vi "以众电机控制.vi"() -> ()   [LabVIEW 2018]
uses:
  Device VIs/Verbal.vi
  <vilib>/Instr/_visa.llb/VISA Configure Serial Port (Instr).vi
panel:
  out "当前位置":i32[](array[numeric])
  in  "小平台X限位":dbl=3000.0 caption="小平台X轴限位/um" min=-8388607.0 max=8388607.0
  in  "设置坐标":bool caption="X jog"
  in  "开始连接":bool
  out "状态":string
  out "执行":bool
  out "OK":bool
  in  "电机":T1(ring)
  in  "结束":bool
  in  "制动":bool
  out "位置信息":i32(listbox)
  out "pic3Left":bool caption="0位"
  out "pic3Right":bool caption="限位"
  out "pic2Left":bool caption="0位"
  out "pic2Right":bool caption="限位"
  out "pic1Left":bool caption="0位"
  out "pic1Right":bool caption="限位"
  out "Z Left":bool caption="0位"
  out "Z Right":bool caption="限位"
  out "Y Left":bool caption="0位"
  out "Y Right":bool caption="限位"
  out "X Lift":bool caption="0位"
  out "X Right":bool caption="限位"
  in  "连续反转":bool
  in  "坐标移动":bool caption="X jog"
  out "设定位置":i32
  in  "坐标":enum16{"位置0", "位置1", "位置2", "位置3"}(ring) caption="位置"
  in  "连续正转":bool
  in  "归0":bool
  in  "启动":bool
  in  "Step":dbl caption="步进\n um" min=-8388607.0 max=8388607.0
  # "电机"
  # "大平台X"
  # "大平台Y"
  # "大平台Z"
  # "小平台X"
  # "小平台Y"
  # "小平台Z"
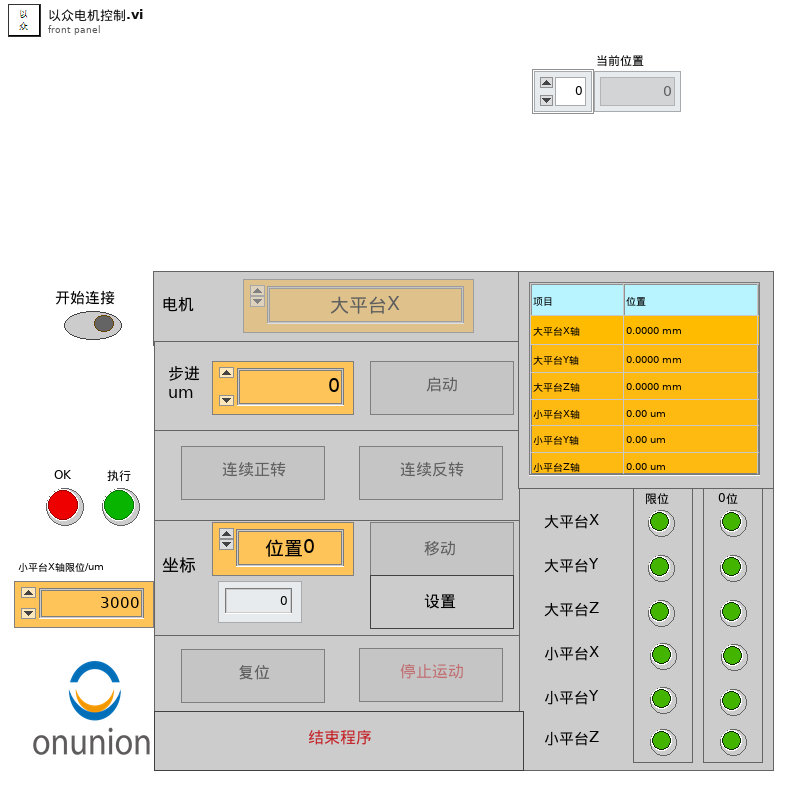
[diagram p1: front panel]
types:
  T1 = enum16{"大平台X", "大平台Y", "大平台Z", "小平台X", "小平台Y", "小平台Z"}
  T2 = enum8{"Enabled", "Disabled", "Disabled and Grayed Out"}
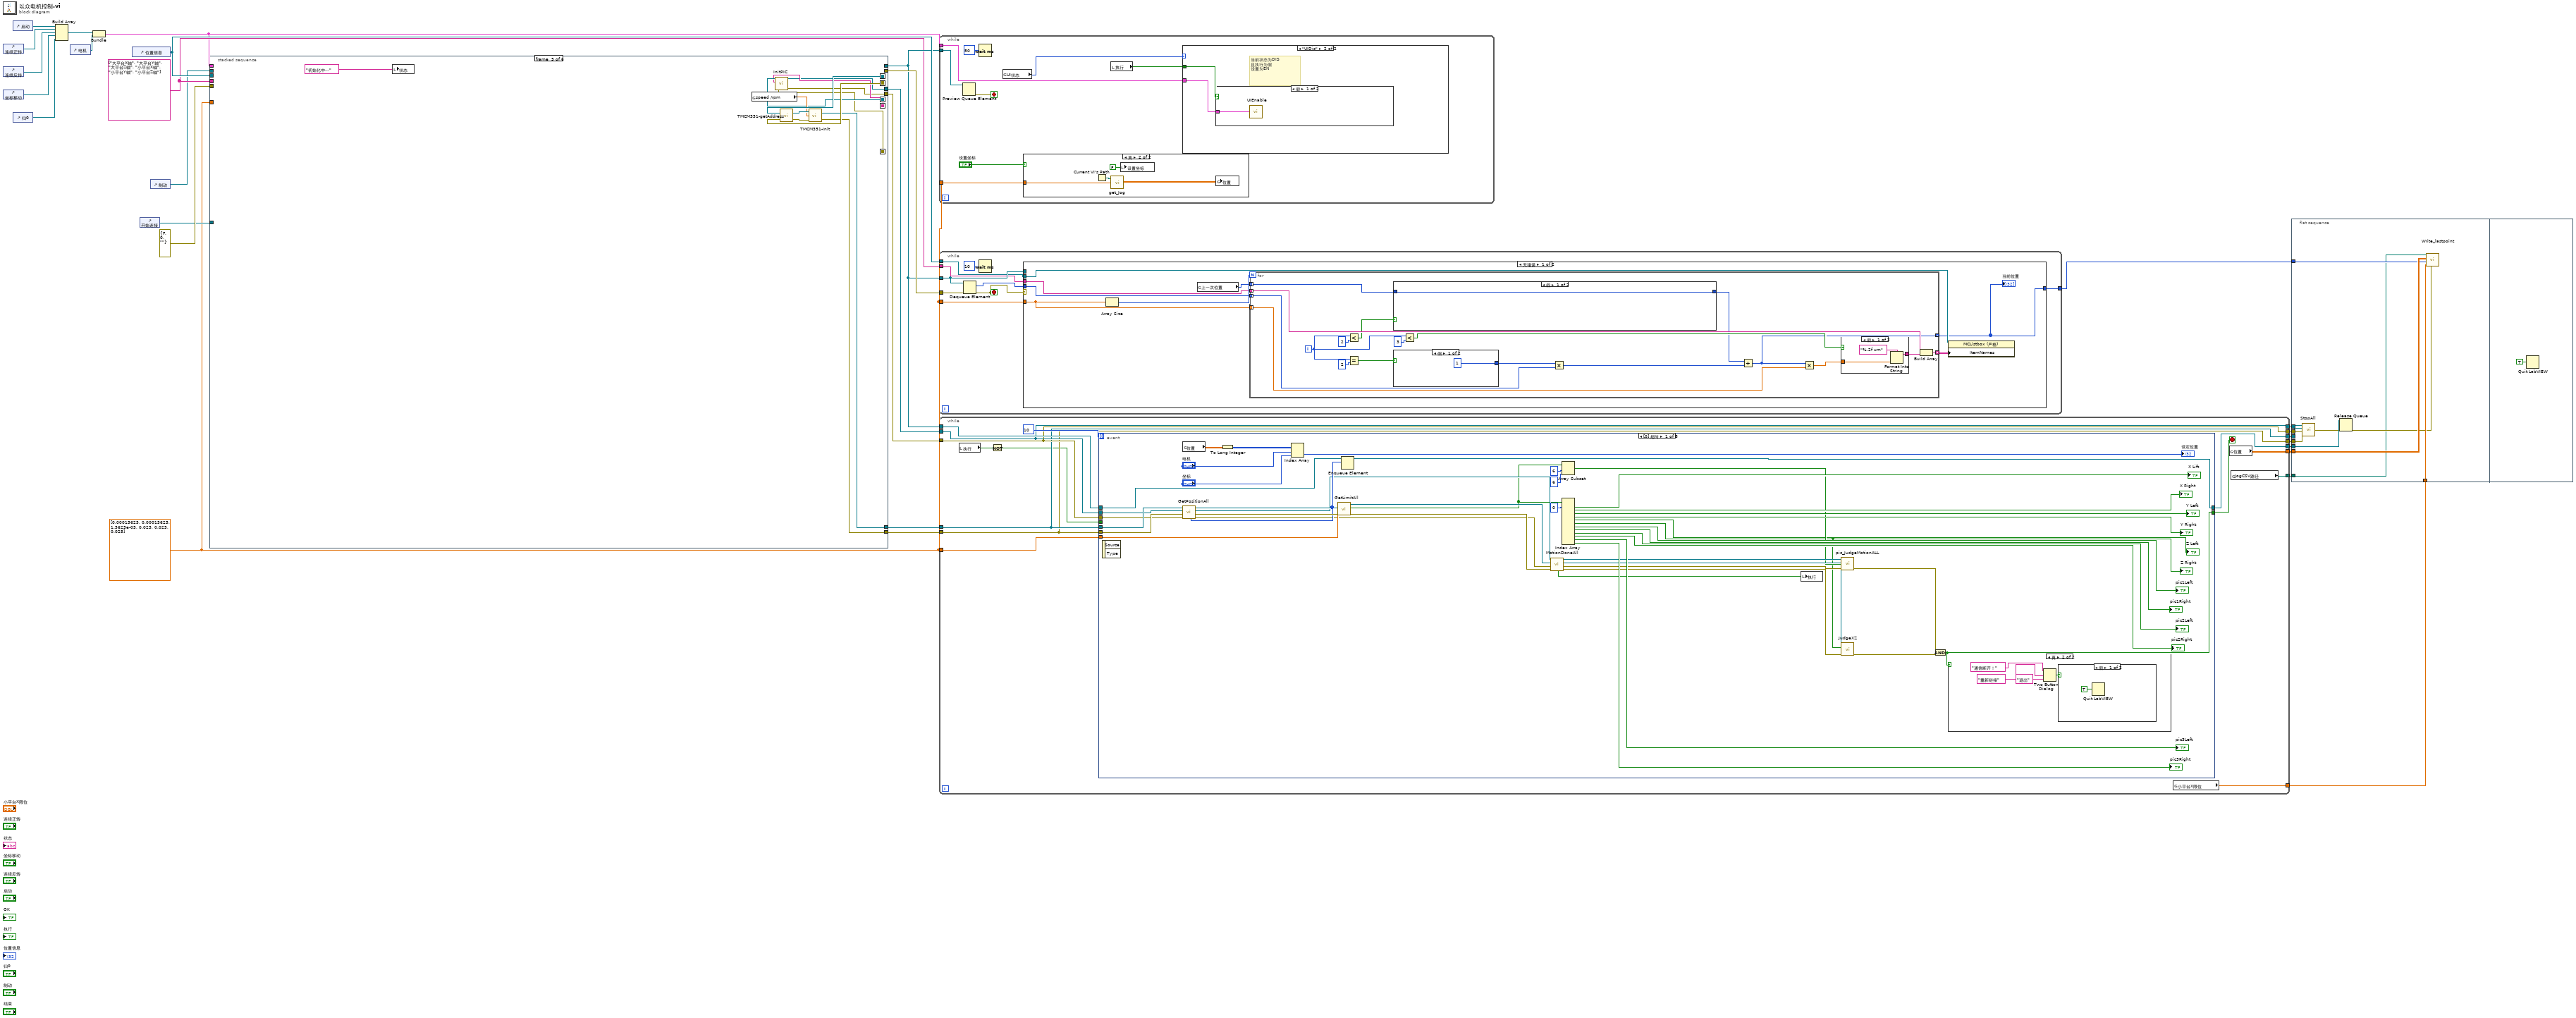
[diagram p0: block diagram]
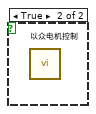
[diagram p3: hidden frame]
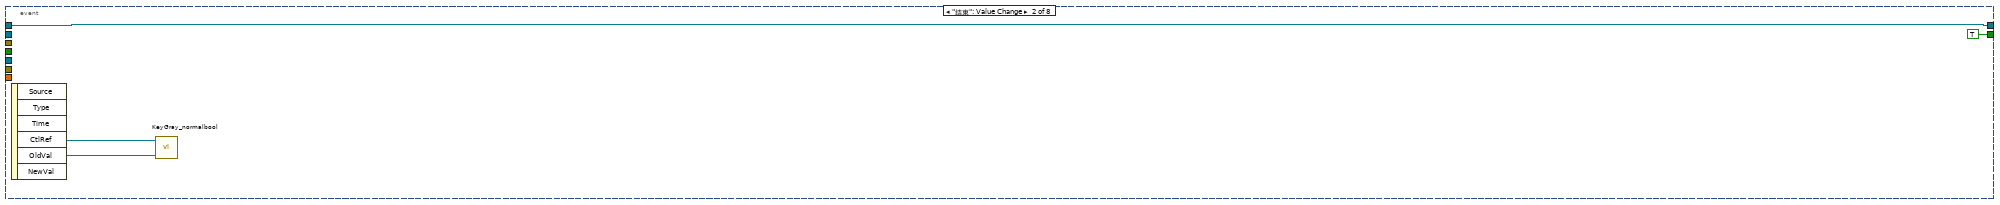
[diagram p4: hidden frame]
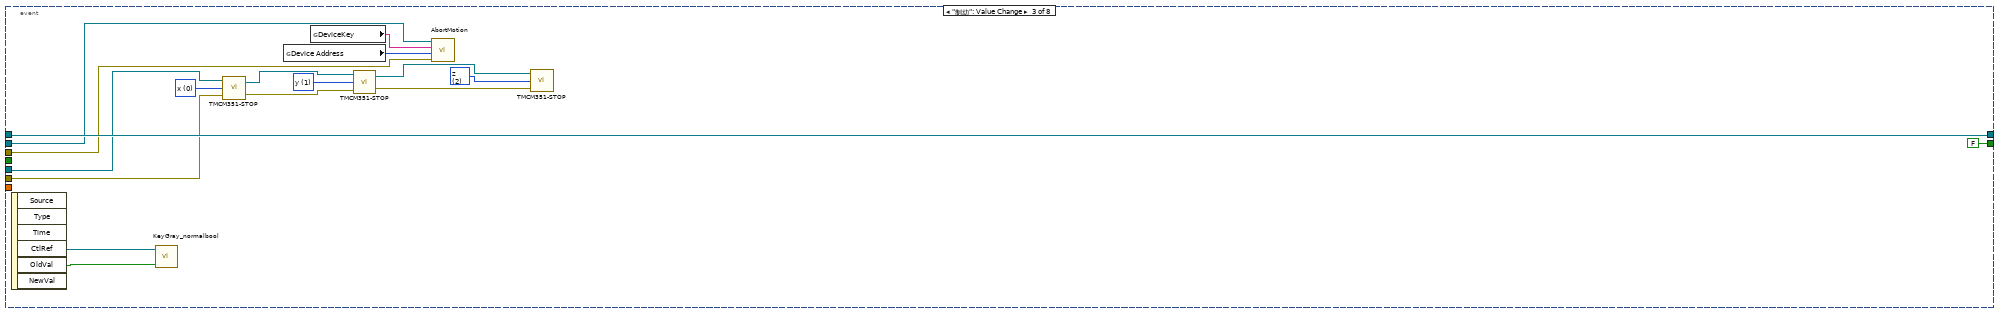
[diagram p5: hidden frame]
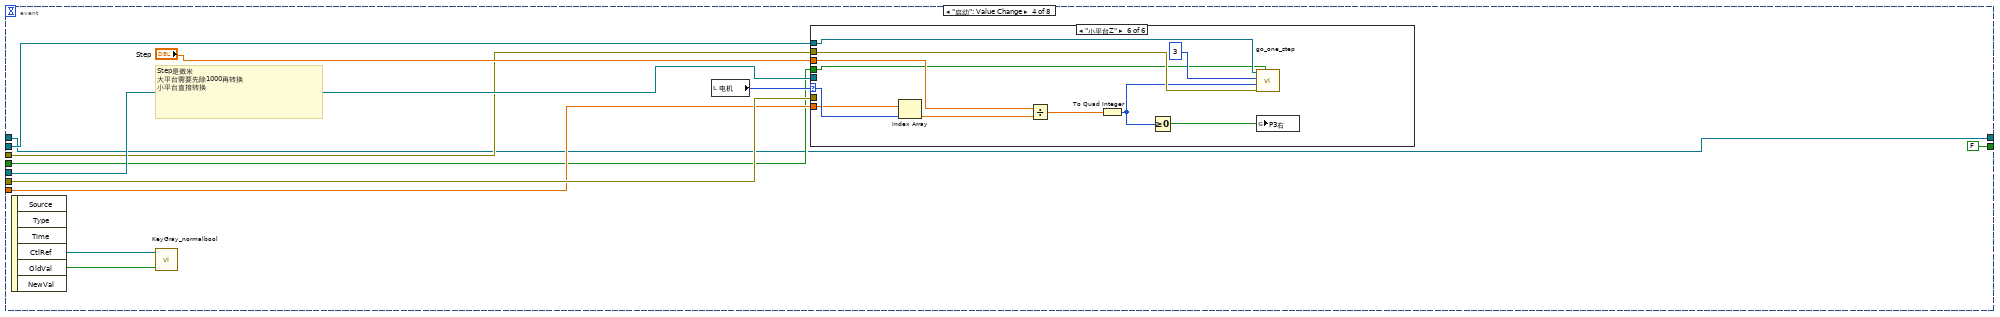
[diagram p6: hidden frame]
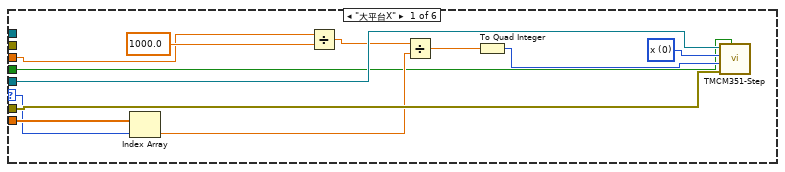
[diagram p7: hidden frame]
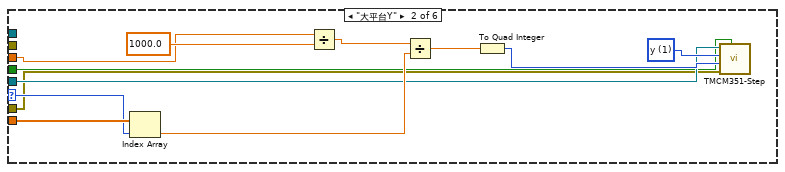
[diagram p8: hidden frame]
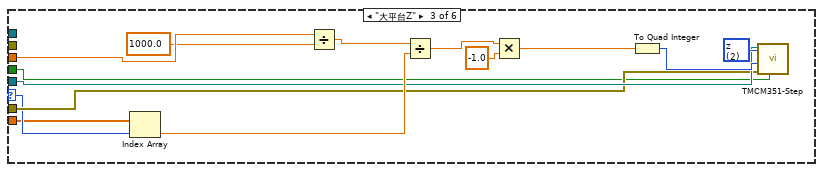
[diagram p9: hidden frame]
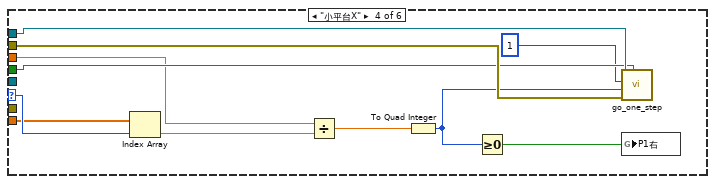
[diagram p10: hidden frame]
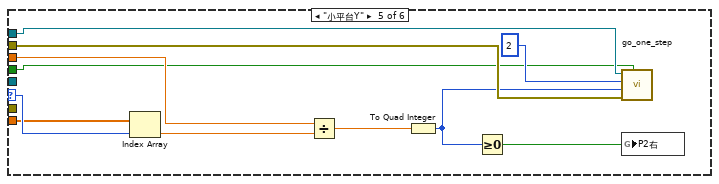
[diagram p11: hidden frame]
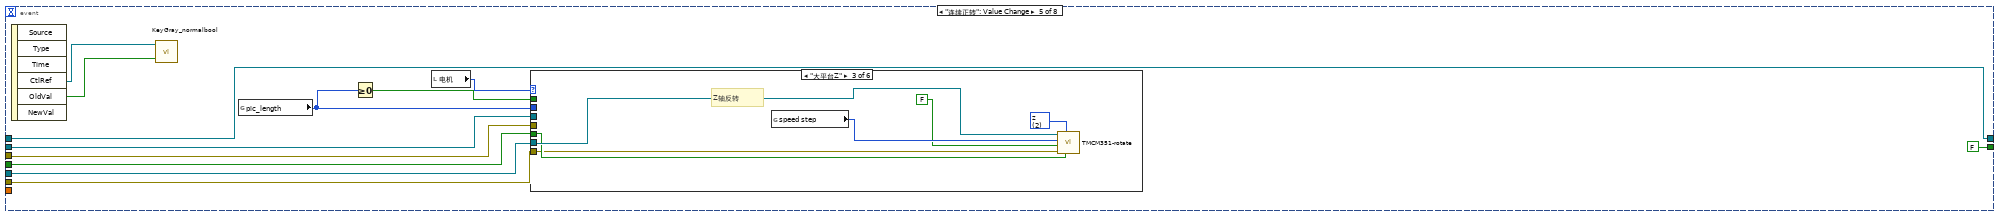
[diagram p12: hidden frame]
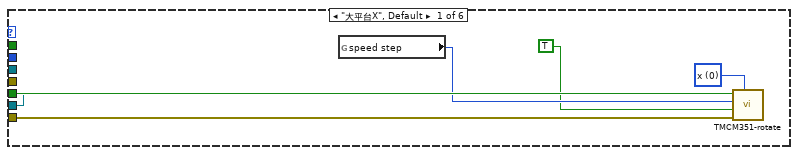
[diagram p13: hidden frame]
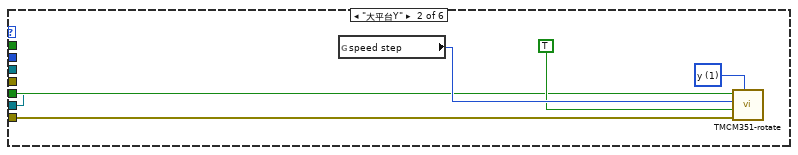
[diagram p14: hidden frame]
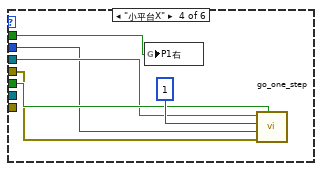
[diagram p15: hidden frame]
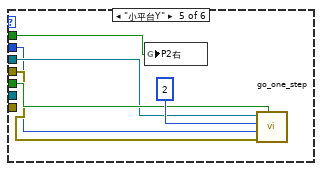
[diagram p16: hidden frame]
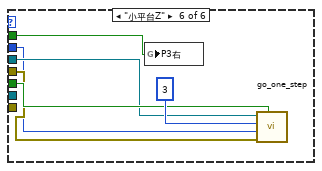
[diagram p17: hidden frame]
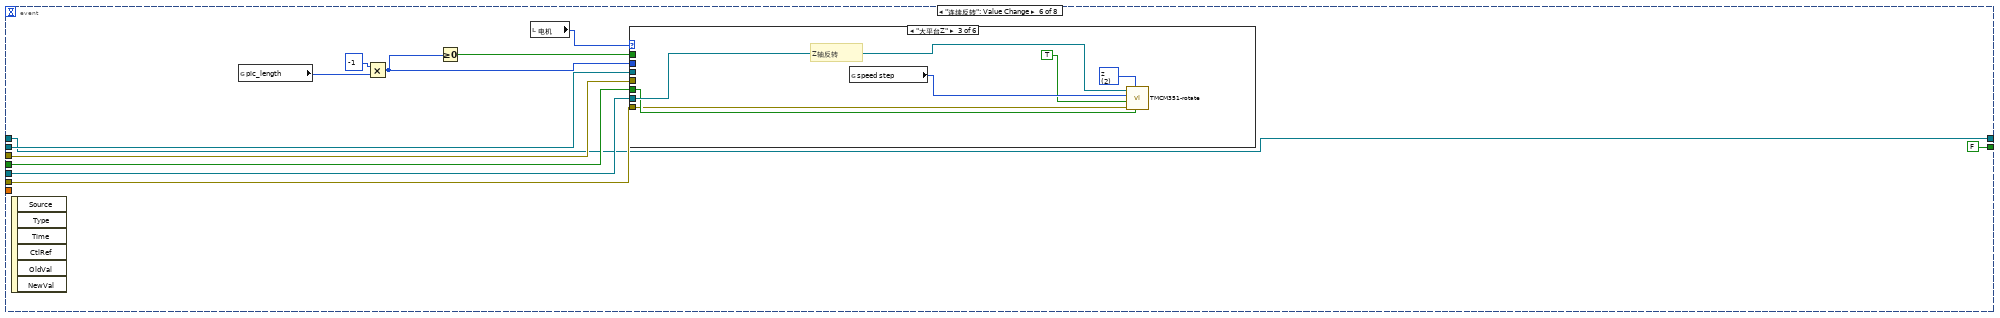
[diagram p18: hidden frame]
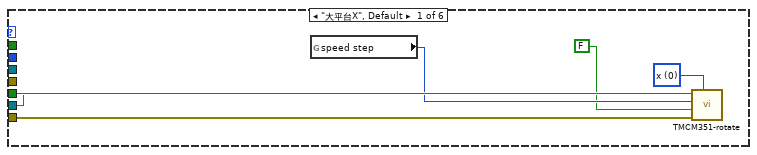
[diagram p19: hidden frame]
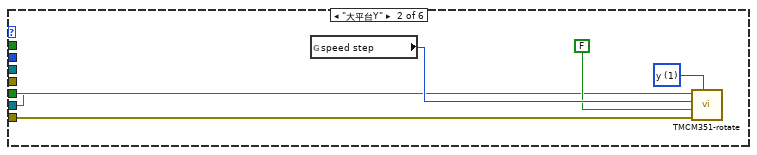
[diagram p20: hidden frame]
diagram:
  w7 = string[] ["大平台X轴", "大平台Y轴", "大平台Z轴", "小平台X轴", "小平台Y轴", "小平台Z轴"]
  w16 = dbl[] [0.00015625, 0.00015625, 1.5625e-05, 0.025, 0.025, 0.025]
  n1 = control-ref of="连续正转"() -> (w27:refnum<vi>)
  n2 = control-ref of="连续反转"() -> (w26:refnum<vi>)
  n3 = control-ref of="坐标移动"() -> (w25:refnum<vi>)
  n4 = control-ref of="启动"() -> (w28:refnum<vi>)
  n5 = control-ref of="归0"() -> (w24:refnum<vi>)
  n6 = Build Array(w28, w27, w26, w25, w24) -> (w4:refnum<vi>[])
  n7 = control-ref of="电机"() -> (w3:refnum<vi>)
  n8 = Bundle(w4, "电机"=w3) -> (w2:cluster{refnum<vi>[], "电机":refnum<vi>})  [unwired: 1 in]
  n9 = control-ref of="位置信息"() -> (w22:refnum<vi>)
  n10 = control-ref of="开始连接"() -> (w23:refnum<vi>)
  n11 = control-ref of="制动"() -> (w6:refnum<vi>)
  n12 = stacked-sequence {
    seq-local: [_ _ _ w75 _ _] -> [_ _ _ _ w107 _]
    seq-local: [_ _ _ w76 _ _] -> [_ _ _ _ w108 _]
    seq-local: [_ _ _ w74 _ _] -> [_ _ _ _ w102 _]
    seq-local: [_ _ _ w73 _ _] -> [_ _ _ _ w101 _]
    seq-local: [_ _ _ w72 _ _] -> [_ _ _ _ w103 _]
    tunnel: w16 -> [_ w46 _ _ _ _]
    tunnel: errorcluster {"status"=FALSE, "code"=0, "source"=""} ("error in (no error)") -> [_ w63 _ w83 _ _]
    tunnel: w22 -> [_ w55 _ _ _ _]
    tunnel: w7 -> [_ w58 _ _ _ _]
    tunnel: w23 -> [w34 _ _ _ _ w121]
    tunnel: [_ _ _ _ w100 _] -> w18
    tunnel: [_ _ _ _ w99 _] -> w17
    tunnel: [_ _ _ _ w98 _] -> w20
    tunnel: [_ _ _ _ w97 _] -> w19
    tunnel: [_ _ _ _ _ w115] -> w8
    tunnel: [_ _ _ _ _ w114] -> w21
    tunnel: w6 -> [w32 _ _ _ _ w112]
    tunnel: w2 -> [w30 _ _ _ _ w110]
    frame #0 {
      n13 = call "UIDisable.vi"("引用簇"=w30) -> ()  [unwired: 1 in]
      n14 = property class="Bool (严格)"(reference=w34, "DisabledEnum"=T2."Enabled" ("禁用")) -> ()  [unwired: 1 in, 2 out]
      n15 = property class="Bool (严格)"(reference=w32, "DisabledEnum"=T2."Disabled and Grayed Out" ("禁用")) -> ()  [unwired: 1 in, 2 out]
    }
    frame #1 {
      w37 = FALSE
      w36 = FALSE
      w38 = FALSE
      w40 = FALSE
      n16 = Current VI's Path() -> (path=w64:path)
      n17 = Array Size(array=w58) -> (size(s)=w57:i32)
      n18 = Index Array(array=w46, index=3 ("索引")) -> (element=w44:dbl)
      n19 = call "get_Jog.vi"("error in (no error)"=w63, "坐标转换"=w46, "路径"=w64) -> ("上次限位"=w35:dbl, "当前位置"=w59:string[], "坐标位置"=w48:dbl[][], "上一次位置"=w47:i32[], "File Out"=w39:path)  [unwired: 1 out]
      n20 = local write "执行"(FALSE ("执行")) -> ()
      n21 = local write "OK"(FALSE ("OK")) -> ()
      n22 = global write "Verbal.vi" "speed /rpm"(10 ("speed step")) -> ()
      n23 = global write "Verbal.vi" "acc pic"(10000 ("acc pic")) -> ()
      n24 = global write "Verbal.vi" "px0?"(w40) -> ()
      n25 = global write "Verbal.vi" "py0?"(w40) -> ()
      n26 = global write "Verbal.vi" "pz0?"(w40) -> ()
      n27 = global write "Verbal.vi" "xz0?"(w40) -> ()
      n28 = local write "Z Left"(w37) -> ()
      n29 = local write "pic1Left"(w37) -> ()
      n30 = local write "pic2Left"(w37) -> ()
      n31 = local write "pic3Left"(w37) -> ()
      n32 = local write "pic2Right"(w36) -> ()
      n33 = local write "pic3Right"(w36) -> ()
      n34 = local write "X Lift"(w36) -> ()
      n35 = local write "Y Left"(w36) -> ()
      n36 = local write "开始连接"(w36) -> ()
      n37 = local write "设置坐标"(w36) -> ()
      n38 = local write "X Right"(w38) -> ()
      n39 = local write "Y Right"(w38) -> ()
      n40 = local write "Z Right"(w38) -> ()
      n41 = local write "pic1Right"(w38) -> ()
      n42 = global write "Verbal.vi" "speed pic"(1000 ("speed pic")) -> ()
      n43 = Build Array("项目", "位置") -> (w62:string[])
      n44 = property on="属性节点" class="MCListbox (严格)"(reference=w55, "ColHdrString"=w62) -> ()  [unwired: 1 in, 2 out]
      n45 = global write "Verbal.vi" "位置"(w48) -> ()
      n46 = global write "Verbal.vi" "上一次位置"(w47) -> ()
      n47 = global write "Verbal.vi" "JogCSV路径"(w39) -> ()
      n48 = global write "Verbal.vi" "小平台X限位"(w35) -> ()
      n49 = local write "小平台X限位"(w35) -> ()
      n50 = for {
        N: w57 -> [_]
        tunnel: w59 -> [w65] mode=indexing
        tunnel: w58 -> [w66] mode=indexing
        tunnel: [w67] -> w56 mode=indexing
        n51 = Build Array(w66, w65) -> (w67:string[])
      }
      n52 = Divide(x=15000.0, y=w44) -> (x/y=w42:dbl)
      n53 = local write "状态"("请点击开始连接" ("状态")) -> ()
      n54 = To Long Integer(number=w42) -> (32bit integer=w41:i32)
      n55 = global write "Verbal.vi" "pic_length"(w41) -> ()
      n56 = property on="属性节点" class="MCListbox (严格)"(reference=w55, "ItemNames"=w56) -> ()  [unwired: 1 in, 2 out]
    }
    frame #2 {
      n57 = flat-sequence {
        frame #0 {
          n58 = while {
            stop <- "开始连接" stop-if-true
            n59 = local read "结束"() -> (w68:bool)
            n60 = Wait (ms)(milliseconds to wait=u32 20 ("等待时间（毫秒）")) -> ()  [unwired: 1 out]
            n61 = Quit LabVIEW(quit? (T)=w68) -> ()
          }
        }
        frame #1 {
          n62 = local write "状态"("查找设备中...." ("状态")) -> ()
        }
      }
    }
    frame #3 {
      n63 = call "InitSingleDevice.vi"("error in (no error)"=w83, "msecDelayForDiscovery"=1000) -> ("error out"=w73:errorcluster, "DeviceKey Out"=w74:string, "CmdLib Out"=w72:refnum<k24>)  [unwired: 3 in]
      n64 = call "findCOM.vi"("error in (no error)"=w83) -> ("错误输出"=w85:errorcluster, "VISA resource out"=w86:refnum<visa-resource-name>)  [unwired: 1 in]
      n65 = String Length(string=w74) -> (length=w82:i32)
      n66 = call-poly "VISA Configure Serial Port"("VISA resource name"=w86, "Enable Termination\nChar (T)"=FALSE ("Enable Termination\nChar (T)"), "baud rate (9600)"=u32 115200, "error in (no error)"=w85) -> ("VISA resource name out"=w79:refnum<visa-resource-name>, "error out"=w78:errorcluster)  [unwired: 10 in]
      n67 = property class="Instr"(reference=w79, error in=w78) -> (reference out=w75:refnum<visa-resource-name>, error out=w76:errorcluster, "Intf Num"=w77:u16)
      n68 = Equal To 0?(x=w82) -> (x = 0?=w81:bool)
      n69 = And(x=w76, y=w81) -> (x .and. y?=w80:bool)
      n70 = case shown="真" w80 {
        tunnel: w74 -> [_ w94]
        tunnel: w77 -> [_ w93]
        frame False {
        }
        frame True {
          n71 = Format Into String(format string="请检查通信和电源\\nCOM:%d;PIC:%s" ("格式字符串"), w93, w94) -> (resulting string=w92:string)  [unwired: 2 in, 1 out]
          n72 = Two Button Dialog(message=w92, 1:"退出" ("F按钮名称（“取消”）"), 2:"重新链接" ("T按钮名称（“确定”）")) -> (T button?=w89:bool)
          n73 = case shown="假" w89 {
            frame False {
              n74 = Quit LabVIEW(quit? (T)=TRUE ("停止？(T)")) -> ()
            }
            frame True {
              n75 = call "以众电机控制.vi"() -> ()  [unwired: 12 in]
            }
          }
        }
      }
    }
    frame #4 {
      n76 = local write "状态"("初始化中..." ("状态")) -> ()
      n77 = global read "Verbal.vi" "speed /rpm"() -> (w104:dbl)
      n78 = call "InitPIC.vi"("error in (no error)"=w101, "DeviceKey In"=w102, "CmdLib In"=w103) -> ("error out"=w99:errorcluster, "CmdLib Out"=w100:refnum<k24>)  [unwired: 1 in, 2 out]
      n79 = call "TMCM351-getAddress.vi"("错误输入"=w108, "com in"=w107) -> ("错误输出"=w105:errorcluster, "com out"=w106:refnum<visa-resource-name>)
      n80 = call "TMCM351-Init.vi"("错误输入"=w105, "Speed /rpm"=w104, "com in"=w106) -> ("错误输出"=w97:errorcluster, "com out"=w98:refnum<visa-resource-name>)
    }
    frame #5 {
      n81 = call "UIEnable.vi"("引用簇"=w110) -> ()  [unwired: 1 in]
      n82 = local write "OK"(TRUE ("OK")) -> ()
      n83 = local write "执行"(FALSE ("执行")) -> ()
      n84 = local write "状态"("欢迎使用" ("状态")) -> ()
      n85 = property class="Bool (严格)"(reference=w112, "DisabledEnum"=T2."Enabled" ("禁用")) -> ()  [unwired: 1 in, 2 out]
      n86 = property class="Bool (严格)"(reference=w121, "DisabledEnum"=T2."Disabled and Grayed Out" ("禁用")) -> ()  [unwired: 1 in, 2 out]
      n87 = Obtain Queue(name (unnamed)="位置消息" ("名称（未命名）"), element data type=i32[] []) -> (queue out=w115:refnum<queue>, error out=w114:errorcluster)  [unwired: 3 in, 1 out]
    }
  }
  n88 = while {
    tunnel: w16 -> [w127]
    tunnel: w2 -> [w124]
    tunnel: w8 -> [w123]
    stop <- w122 stop-if-true
    n89 = Preview Queue Element(queue=w123) -> (error out=w122:errorcluster)  [unwired: 2 in, 3 out]
    n90 = Wait (ms)(milliseconds to wait=u32 50 ("等待时间（毫秒）")) -> ()  [unwired: 1 out]
    n91 = global read "Verbal.vi" "UI状态"() -> (w126:enum16{"UIEn", "UIDis"})
    n92 = case shown="真" "设置坐标" {
      tunnel: w127 -> [_ w137]
      frame False {
      }
      frame True {
        n93 = Current VI's Path() -> (path=w138:path)
        n94 = call "get_Jog.vi"("坐标转换"=w137, "路径"=w138) -> ("坐标位置"=w136:dbl[][])  [unwired: 1 in, 5 out]
        n95 = local write "设置坐标"(FALSE ("设置坐标")) -> ()
        n96 = global write "Verbal.vi" "位置"(w136) -> ()
      }
    }
    n97 = local read "执行"() -> (w125:bool)
    n98 = case shown="\"UIDis\"" w126 {
      tunnel: w124 -> [w131 w134]
      tunnel: w125 -> [w130 w133]
      frame "UIEn", Default {
        # "当前状态为EN\n且执行为真\n设置为Dis"
        n99 = case shown="真" w130 {
          tunnel: w131 -> [_ w132]
          frame False {
          }
          frame True {
            n100 = call "UIDisable.vi"("引用簇"=w132) -> ()  [unwired: 1 in]
          }
        }
      }
      frame "UIDis" {
        # "当前状态为DIS\n且执行为假\n设置为EN"
        n101 = case shown="假" w133 {
          tunnel: w134 -> [w135 _]
          frame False {
            n102 = call "UIEnable.vi"("引用簇"=w135) -> ()  [unwired: 1 in]
          }
          frame True {
          }
        }
      }
    }
  }
  n103 = while {
    tunnel: w8 -> [w148]
    tunnel: w21 -> [w141]
    tunnel: w16 -> [w147]
    tunnel: w7 -> [w146]
    tunnel: w22 -> [w145]
    tunnel: [w144] -> w5
    stop <- w140 stop-if-true
    n104 = Dequeue Element(queue=w148, error in (no error)=w141) -> (element=w142:i32[], error out=w140:errorcluster)  [unwired: 1 in, 2 out]
    n105 = Wait (ms)(milliseconds to wait=u32 10 ("等待时间（毫秒）")) -> ()  [unwired: 1 out]
    n106 = case shown="无错误" w140 {
      tunnel: w148 -> [_ _]
      tunnel: w147 -> [w156 _]
      tunnel: w146 -> [w154 _]
      tunnel: w145 -> [w152 _]
      tunnel: [w149 w185] -> w144
      tunnel: w142 -> [w150 _]
      frame No Error {
        n107 = Array Size(array=w156) -> (size(s)=w155:i32)
        n108 = global read "Verbal.vi" "上一次位置"() -> (w151:i32[])
        n109 = for {
          N: w155 -> [_]
          tunnel: w156 -> [w174] mode=indexing
          tunnel: w154 -> [w171] mode=indexing
          tunnel: [w169] -> w153 mode=indexing
          tunnel: w151 -> [w166] mode=indexing
          tunnel: [w165] -> w149 mode=indexing
          tunnel: w150 -> [w159] mode=indexing
          i -> [w164]
          n110 = Less?(x=w164, y=2) -> (x < y?=w167:bool)
          n111 = Equal?(x=w164, y=2) -> (x = y?=w161:bool)
          n112 = case shown="假" w167 {
            tunnel: [w177 0] -> w157
            tunnel: w166 -> [w177 _]
            frame False {
            }
            frame True {
              # "小于2是大平台XY\n已经写入了不用修正"
            }
          }
          n113 = case shown="假" w161 {
            tunnel: [1 -1] -> w162
            frame False {
            }
            frame True {
            }
          }
          n114 = Less?(x=w164, y=3) -> (x < y?=w172:bool)
          n115 = Multiply(x=w162, y=w159) -> (x*y=w158:i32)
          n116 = Add(x=w157, y=w158) -> (x+y=w165:i32)
          n117 = Multiply(x=w165, y=w174) -> (x*y=w160:dbl)
          n118 = case shown="假" w172 {
            tunnel: w160 -> [w179 w182]
            tunnel: [w180 w183] -> w170
            frame False {
              n119 = Format Into String(format string="%.2f um" ("格式字符串"), w179) -> (resulting string=w180:string)  [unwired: 2 in, 1 out]
            }
            frame True {
              n120 = Format Into String(format string="%.4f mm" ("格式字符串"), w182) -> (resulting string=w183:string)  [unwired: 2 in, 1 out]
            }
          }
          n121 = Build Array(w171, w170) -> (w169:string[])
        }
        "当前位置" <- w149
        n122 = property on="属性节点" class="MCListbox (严格)"(reference=w152, "ItemNames"=w153) -> ()  [unwired: 1 in, 2 out]
      }
      frame Error {
        n123 = local read "当前位置"() -> (w185:i32[])
      }
    }
  }
  n124 = while {
    tunnel: w8 -> [w198]
    tunnel: w20 -> [w192]
    tunnel: w19 -> [w191]
    tunnel: w18 -> [w194]
    tunnel: w17 -> [w193]
    tunnel: w16 -> [w197]
    tunnel: [w196] -> w15
    tunnel: [w194] -> w14
    tunnel: [w193] -> w13
    tunnel: [w192] -> w12
    tunnel: [w191] -> w11
    tunnel: [w188] -> w10
    tunnel: [w187] -> w9
    tunnel: [w186] -> w1
    stop <- w195 stop-if-true
    n125 = local read "执行"() -> (w190:bool)
    n126 = Not(x=w190) -> (.not. x?=w189:bool)
    n127 = event shown="[0] 超时" {
      selector: _ -> [_ _ _ _ _ _ _ _]
      dyn-events: _ -> [_ _ _ _ _ _ _ _]
      timeout: 10 -> [_ _ _ _ _ _ _ _]
      tunnel: w192 -> [w238 _ w257 w280 w360 w408 w457 w513]
      tunnel: w191 -> [w237 _ w256 w279 w359 w407 w456 w514]
      tunnel: w194 -> [w236 _ w254 w276 w358 w409 w458 w511]
      tunnel: w193 -> [w235 _ w253 w275 w355 w410 w459 w510]
      tunnel: w198 -> [w234 w252 w267 w271 w354 w402 w450 w500]
      tunnel: w197 -> [w230 _ _ w277 _ _ _ w509]
      tunnel: [w210 w252 w267 w271 w354 w402 w450 w500] -> w196
      tunnel: [w209 TRUE FALSE FALSE FALSE FALSE FALSE FALSE] -> w195
      tunnel: w189 -> [_ _ _ w274 w361 w403 w460 w512]
      event Timeout {
        n128 = event-data() -> ()  [unwired: 1 in, 2 out]
        n129 = global read "Verbal.vi" "位置"() -> (w243:dbl[][])
        n130 = call "GetPositionAll.vi"("PicError"=w235, "StepError"=w237, "CmdLib In"=w236, "com in"=w238) -> ("PicErrorOut"=w215:errorcluster, "StepError"=w232:errorcluster, "CmdLib Out"=w216:refnum<k24>, "com out"=w233:refnum<visa-resource-name>, "PositionOut"=w231:i32[])  [unwired: 3 in]
        n131 = To Long Integer(number=w243) -> (32bit integer=w242:i32[][])
        n132 = Index Array(array=w242, index (row)="电机", index (col)="坐标") -> (element=→"设定位置":i32)
        n133 = call "GetLimitAll.vi"("StepError"=w232, "坐标变换"=w230, "PositionIn"=w231, "com in"=w233) -> ("StepErrorOut"=w217:errorcluster, "限位输出"=w206:bool[], "com out"=w218:refnum<visa-resource-name>)  [unwired: 1 in]
        n134 = Enqueue Element(queue=w234, element=w231) -> (queue out=w210:refnum<queue>)  [unwired: 2 in, 2 out]
        n135 = call "MotionDoneAll.vi"("StepError"=w217, "PicError"=w215, "com in"=w218, "CmdLib In"=w216) -> ("StepErrorOut"=w212:errorcluster, "PicErrorOut"=w207:errorcluster, "com out"=w213:refnum<visa-resource-name>, "CmdLib Out"=w208:refnum<k24>, "执行"=w214:bool)  [unwired: 3 in]
        n136 = Array Subset(array=w206, index=6 ("索引"), length=6 ("长度")) -> (w203:bool[])
        n137 = Index Array(array=w206, index #1=0 ("索引")) -> (element #1=→"X Lift":bool, element #2=→"X Right":bool, element #3=→"Y Left":bool, element #4=→"Y Right":bool, element #5=→"Z Left":bool, element #6=w200:bool, element #7=→"pic1Left":bool, element #8=→"pic1Right":bool, element #9=→"pic2Left":bool, element #10=→"pic2Right":bool, element #11=→"pic3Left":bool, element #12=→"pic3Right":bool)  [unwired: 11 in]
        "Z Right" <- w200
        n138 = local write "执行"(w214) -> ()
        n139 = call "pic_JudgeMotionALL.vi"("error in)"=w207, "Limit"=w203, "CmdLib In"=w208) -> ("error out"=w202:errorcluster)  [unwired: 1 in, 1 out]
        n140 = call "JudgeXZ.vi"("错误输入"=w212, "Z Right Limit"=w200, "com in"=w213) -> ("错误输出"=w211:errorcluster)  [unwired: 7 in, 1 out]
        n141 = And(x=w202, y=w211) -> (x .and. y?=w209:bool)
        n142 = case shown="真" w209 {
          frame False {
          }
          frame True {
            n143 = Two Button Dialog(message="通信断开！" ("消息"), 1:"退出" ("F按钮名称（“取消”）"), 2:"重新链接" ("T按钮名称（“确定”）")) -> (T button?=w245:bool)
            n144 = case shown="假" w245 {
              frame False {
                n145 = Quit LabVIEW(quit? (T)=TRUE ("停止？(T)")) -> ()
              }
              frame True {
                n146 = call "以众电机控制.vi"() -> ()  [unwired: 12 in]
              }
            }
          }
        }
      }
      event "结束": Value Change {
        n147 = event-data() -> ("CtlRef"=w250:refnum<vi>, "OldVal"=w249:bool)  [unwired: 1 in, 4 out]
        n148 = call "KeyGray_normalbool.vi"("OldVal"=w249, "引用"=w250) -> ()  [unwired: 2 in]
      }
      event "制动": Value Change {
        w255 = u8 0 items=["x", "y", "z"] ("motor")
        w259 = u8 2 items=["x", "y", "z"] ("motor")
        w262 = u8 1 items=["x", "y", "z"] ("motor")
        n149 = event-data() -> ("CtlRef"=w269:refnum<vi>, "OldVal"=w268:bool)  [unwired: 1 in, 4 out]
        n150 = call "KeyGray_normalbool.vi"("OldVal"=w268, "引用"=w269) -> ()  [unwired: 2 in]
        n151 = call "TMCM351-STOP.vi"("错误输入"=w256, "motor"=w255, "com in"=w257) -> ("错误输出"=w263:errorcluster, "com out"=w264:refnum<visa-resource-name>)
        n152 = global read "Verbal.vi" "Device Address"() -> (w258:i32)
        n153 = global read "Verbal.vi" "DeviceKey"() -> (w265:string)
        n154 = call "TMCM351-STOP.vi"("错误输入"=w263, "motor"=w262, "com in"=w264) -> ("错误输出"=w260:errorcluster, "com out"=w261:refnum<visa-resource-name>)
        n155 = call "AbortMotion.vi"("error in (no error)"=w253, "Device Address In"=w258, "DeviceKey In"=w265, "CmdLib In"=w254) -> ()  [unwired: 4 out]
        n156 = call "TMCM351-STOP.vi"("错误输入"=w260, "motor"=w259, "com in"=w261) -> ()  [unwired: 2 out]
      }
      event "启动": Value Change {
        # "Step是微米\n大平台需要先除1000再转换\n小平台直接转换"
        n157 = event-data() -> ("CtlRef"=w273:refnum<vi>, "OldVal"=w272:bool)  [unwired: 1 in, 4 out]
        n158 = call "KeyGray_normalbool.vi"("OldVal"=w272, "引用"=w273) -> ()  [unwired: 2 in]
        n159 = local read "电机"() -> (w281:T1)
        n160 = case shown="\"小平台Z\"" w281 {
          selector: w281 -> [w289 w300 w314 w325 w339 w348]
          tunnel: w280 -> [w293 w299 w316 _ _ _]
          tunnel: w279 -> [w292 w298 w315 _ _ _]
          tunnel: "Step" -> [w283 w295 w311 w324 w338 w347]
          tunnel: w277 -> [w290 w301 w313 w323 w337 w346]
          tunnel: w274 -> [w285 w297 w312 w328 w334 w345]
          tunnel: w276 -> [_ _ _ w330 w336 w350]
          tunnel: w275 -> [_ _ _ w329 w335 w349]
          frame "大平台X" {
            w291 = u8 0 items=["x", "y", "z"] ("motor")
            n161 = Index Array(array=w290, index=w289) -> (element=w288:dbl)
            n162 = Divide(x=w283, y=1000.0) -> (x/y=w282:dbl)
            n163 = Divide(x=w282, y=w288) -> (x/y=w287:dbl)
            n164 = To Quad Integer(1:w287) -> (0:w286:i64)
            n165 = call "TMCM351-Step.vi"("执行完毕"=w285, "错误输入"=w292, "Step"=w286, "motor"=w291, "com in"=w293) -> ()  [unwired: 2 in, 2 out]
          }
          frame "大平台Y" {
            w305 = u8 1 items=["x", "y", "z"] ("motor")
            n166 = Index Array(array=w301, index=w300) -> (element=w304:dbl)
            n167 = Divide(x=w295, y=1000.0) -> (x/y=w294:dbl)
            n168 = Divide(x=w294, y=w304) -> (x/y=w303:dbl)
            n169 = To Quad Integer(1:w303) -> (0:w302:i64)
            n170 = call "TMCM351-Step.vi"("执行完毕"=w297, "错误输入"=w298, "Step"=w302, "motor"=w305, "com in"=w299) -> ()  [unwired: 2 in, 2 out]
          }
          frame "大平台Z" {
            w319 = u8 2 items=["x", "y", "z"] ("motor")
            n171 = Index Array(array=w313, index=w314) -> (element=w318:dbl)
            n172 = Divide(x=w311, y=1000.0) -> (x/y=w310:dbl)
            n173 = Divide(x=w310, y=w318) -> (x/y=w308:dbl)
            n174 = Multiply(x=w308, y=-1.0) -> (x*y=w306:dbl)
            n175 = To Quad Integer(1:w306) -> (0:w317:i64)
            n176 = call "TMCM351-Step.vi"("执行完毕"=w312, "错误输入"=w315, "Step"=w317, "motor"=w319, "com in"=w316) -> ()  [unwired: 2 in, 2 out]
          }
          frame "小平台X" {
            n177 = Index Array(array=w323, index=w325) -> (element=w326:dbl)
            n178 = Divide(x=w324, y=w326) -> (x/y=w322:dbl)
            n179 = To Quad Integer(1:w322) -> (0:w321:i64)
            n180 = Greater Or Equal To 0?(x=w321) -> (x >= 0?=w320:bool)
            n181 = call "go_one_step.vi"("执行完毕"=w328, "error in"=w329, "Step"=w321, "Motor"=1, "CmdLib In"=w330) -> ()  [unwired: 1 in, 3 out]
            n182 = global write "Verbal.vi" "P1右"(w320) -> ()
          }
          frame "小平台Y" {
            n183 = Index Array(array=w337, index=w339) -> (element=w340:dbl)
            n184 = Divide(x=w338, y=w340) -> (x/y=w333:dbl)
            n185 = To Quad Integer(1:w333) -> (0:w331:i64)
            n186 = Greater Or Equal To 0?(x=w331) -> (x >= 0?=w332:bool)
            n187 = call "go_one_step.vi"("执行完毕"=w334, "error in"=w335, "Step"=w331, "Motor"=2, "CmdLib In"=w336) -> ()  [unwired: 1 in, 3 out]
            n188 = global write "Verbal.vi" "P2右"(w332) -> ()
          }
          frame "小平台Z" {
            n189 = Index Array(array=w346, index=w348) -> (element=w351:dbl)
            n190 = Divide(x=w347, y=w351) -> (x/y=w344:dbl)
            n191 = To Quad Integer(1:w344) -> (0:w342:i64)
            n192 = Greater Or Equal To 0?(x=w342) -> (x >= 0?=w343:bool)
            n193 = call "go_one_step.vi"("执行完毕"=w345, "error in"=w349, "Step"=w342, "Motor"=3, "CmdLib In"=w350) -> ()  [unwired: 1 in, 3 out]
            n194 = global write "Verbal.vi" "P3右"(w343) -> ()
          }
        }
      }
      event "连续正转": Value Change {
        n195 = event-data() -> ("CtlRef"=w364:refnum<vi>, "OldVal"=w363:bool)  [unwired: 1 in, 4 out]
        n196 = call "KeyGray_normalbool.vi"("OldVal"=w363, "引用"=w364) -> ()  [unwired: 2 in]
        n197 = global read "Verbal.vi" "pic_length"() -> (w356:i32)
        n198 = Greater Or Equal To 0?(x=w356) -> (x >= 0?=w357:bool)
        n199 = local read "电机"() -> (w362:T1)
        n200 = case shown="\"大平台Z\"" w362 {
          tunnel: w361 -> [w369 w373 w378 w387 w393 w399]
          tunnel: w360 -> [w368 w372 w379 _ _ _]
          tunnel: w359 -> [w365 w371 w377 _ _ _]
          tunnel: w358 -> [_ _ _ w386 w391 w397]
          tunnel: w357 -> [_ _ _ w385 w389 w395]
          tunnel: w356 -> [_ _ _ w384 w390 w396]
          tunnel: w355 -> [_ _ _ w383 w392 w398]
          frame "大平台X", Default {
            w370 = u8 0 items=["x", "y", "z"] ("motor")
            n201 = global read "Verbal.vi" "speed step"() -> (w367:i32)
            n202 = call "TMCM351-rotate.vi"("执行？"=w369, "motor"=w370, "错误输入"=w365, "正转？"=TRUE, "Speed"=w367, "com in"=w368) -> ()  [unwired: 2 in, 2 out]
          }
          frame "大平台Y" {
            w376 = u8 1 items=["x", "y", "z"] ("motor")
            n203 = global read "Verbal.vi" "speed step"() -> (w375:i32)
            n204 = call "TMCM351-rotate.vi"("执行？"=w373, "motor"=w376, "错误输入"=w371, "正转？"=TRUE, "Speed"=w375, "com in"=w372) -> ()  [unwired: 2 in, 2 out]
          }
          frame "大平台Z" {
            w382 = u8 2 items=["x", "y", "z"] ("motor")
            # "Z轴反转"
            n205 = global read "Verbal.vi" "speed step"() -> (w381:i32)
            n206 = call "TMCM351-rotate.vi"("执行？"=w378, "motor"=w382, "错误输入"=w377, "正转？"=FALSE, "Speed"=w381, "com in"=w379) -> ()  [unwired: 2 in, 2 out]
          }
          frame "小平台X" {
            n207 = global write "Verbal.vi" "P1右"(w385) -> ()
            n208 = call "go_one_step.vi"("执行完毕"=w387, "error in"=w383, "Step"=w384, "Motor"=1, "CmdLib In"=w386) -> ()  [unwired: 1 in, 3 out]
          }
          frame "小平台Y" {
            n209 = global write "Verbal.vi" "P2右"(w389) -> ()
            n210 = call "go_one_step.vi"("执行完毕"=w393, "error in"=w392, "Step"=w390, "Motor"=2, "CmdLib In"=w391) -> ()  [unwired: 1 in, 3 out]
          }
          frame "小平台Z" {
            n211 = global write "Verbal.vi" "P3右"(w395) -> ()
            n212 = call "go_one_step.vi"("执行完毕"=w399, "error in"=w398, "Step"=w396, "Motor"=3, "CmdLib In"=w397) -> ()  [unwired: 1 in, 3 out]
          }
        }
      }
      event "连续反转": Value Change {
        n213 = event-data() -> ()  [unwired: 1 in, 6 out]
        n214 = global read "Verbal.vi" "pic_length"() -> (w411:i32)
        n215 = Multiply(x=-1, y=w411) -> (x*y=w405:i32)
        n216 = Greater Or Equal To 0?(x=w405) -> (x >= 0?=w412:bool)
        n217 = local read "电机"() -> (w406:T1)
        n218 = case shown="\"大平台Z\"" w406 {
          tunnel: w403 -> [w417 w421 w426 w435 w441 w447]
          tunnel: w408 -> [w416 w420 w427 _ _ _]
          tunnel: w407 -> [w413 w419 w425 _ _ _]
          tunnel: w409 -> [_ _ _ w434 w439 w445]
          tunnel: w412 -> [_ _ _ w433 w437 w443]
          tunnel: w405 -> [_ _ _ w432 w438 w444]
          tunnel: w410 -> [_ _ _ w431 w440 w446]
          frame "大平台X", Default {
            w418 = u8 0 items=["x", "y", "z"] ("motor")
            n219 = global read "Verbal.vi" "speed step"() -> (w415:i32)
            n220 = call "TMCM351-rotate.vi"("执行？"=w417, "motor"=w418, "错误输入"=w413, "正转？"=FALSE, "Speed"=w415, "com in"=w416) -> ()  [unwired: 2 in, 2 out]
          }
          frame "大平台Y" {
            w424 = u8 1 items=["x", "y", "z"] ("motor")
            n221 = global read "Verbal.vi" "speed step"() -> (w423:i32)
            n222 = call "TMCM351-rotate.vi"("执行？"=w421, "motor"=w424, "错误输入"=w419, "正转？"=FALSE, "Speed"=w423, "com in"=w420) -> ()  [unwired: 2 in, 2 out]
          }
          frame "大平台Z" {
            w430 = u8 2 items=["x", "y", "z"] ("motor")
            # "Z轴反转"
            n223 = global read "Verbal.vi" "speed step"() -> (w429:i32)
            n224 = call "TMCM351-rotate.vi"("执行？"=w426, "motor"=w430, "错误输入"=w425, "正转？"=TRUE, "Speed"=w429, "com in"=w427) -> ()  [unwired: 2 in, 2 out]
          }
          frame "小平台X" {
            n225 = global write "Verbal.vi" "P1右"(w433) -> ()
            n226 = call "go_one_step.vi"("执行完毕"=w435, "error in"=w431, "Step"=w432, "Motor"=1, "CmdLib In"=w434) -> ()  [unwired: 1 in, 3 out]
          }
          frame "小平台Y" {
            n227 = global write "Verbal.vi" "P2右"(w437) -> ()
            n228 = call "go_one_step.vi"("执行完毕"=w441, "error in"=w440, "Step"=w438, "Motor"=2, "CmdLib In"=w439) -> ()  [unwired: 1 in, 3 out]
          }
          frame "小平台Z" {
            n229 = global write "Verbal.vi" "P3右"(w443) -> ()
            n230 = call "go_one_step.vi"("执行完毕"=w447, "error in"=w446, "Step"=w444, "Motor"=3, "CmdLib In"=w445) -> ()  [unwired: 1 in, 3 out]
          }
        }
      }
      event "归0": Value Change {
        n231 = event-data() -> ("CtlRef"=w462:refnum<vi>, "OldVal"=w461:bool)  [unwired: 1 in, 4 out]
        n232 = call "KeyGray_normalbool.vi"("OldVal"=w461, "引用"=w462) -> ()  [unwired: 2 in]
        n233 = global read "Verbal.vi" "pic_length"() -> (w454:i32)
        n234 = Multiply(x=-1, y=w454) -> (x*y=w452:i32)
        n235 = Greater Or Equal To 0?(x=w452) -> (x >= 0?=w451:bool)
        n236 = local read "电机"() -> (w455:T1)
        n237 = case shown="\"大平台Z\"" w455 {
          tunnel: w460 -> [w464 w469 w473 w483 w490 w497]
          tunnel: w457 -> [w465 w468 w474 _ _ _]
          tunnel: w456 -> [w463 w467 w472 _ _ _]
          tunnel: w458 -> [_ _ _ w482 w488 w495]
          tunnel: w459 -> [_ _ _ w481 w489 w496]
          tunnel: w452 -> [_ _ _ w480 w487 w494]
          tunnel: w451 -> [_ _ _ w479 w486 w493]
          frame "大平台X", Default {
            w466 = u8 0 items=["x", "y", "z"] ("motor")
            n238 = call "TMCM1021_goRef.vi"("错误输入"=w463, "motor"=w466, "执行？"=w464, "com in"=w465) -> ()  [unwired: 2 out]
          }
          frame "大平台Y" {
            w470 = u8 1 items=["x", "y", "z"] ("motor")
            n239 = call "TMCM1021_goRef.vi"("错误输入"=w467, "motor"=w470, "执行？"=w469, "com in"=w468) -> ()  [unwired: 2 out]
          }
          frame "大平台Z" {
            w477 = u8 2 items=["x", "y", "z"] ("motor")
            # "Z轴反转\n记录0位"
            n240 = global write "Verbal.vi" "xz0?"(TRUE ("xz0?")) -> ()
            n241 = global read "Verbal.vi" "speed step"() -> (w476:i32)
            n242 = call "TMCM351-rotate.vi"("执行？"=w473, "motor"=w477, "错误输入"=w472, "正转？"=TRUE, "Speed"=w476, "com in"=w474) -> ()  [unwired: 2 in, 2 out]
          }
          frame "小平台X" {
            n243 = global write "Verbal.vi" "P1右"(w479) -> ()
            n244 = global write "Verbal.vi" "px0?"(TRUE ("px0?")) -> ()
            n245 = call "go_one_step.vi"("执行完毕"=w483, "error in"=w481, "Step"=w480, "Motor"=1, "CmdLib In"=w482) -> ()  [unwired: 1 in, 3 out]
          }
          frame "小平台Y" {
            n246 = global write "Verbal.vi" "P2右"(w486) -> ()
            n247 = global write "Verbal.vi" "py0?"(TRUE ("py0?")) -> ()
            n248 = call "go_one_step.vi"("执行完毕"=w490, "error in"=w489, "Step"=w487, "Motor"=2, "CmdLib In"=w488) -> ()  [unwired: 1 in, 3 out]
          }
          frame "小平台Z" {
            n249 = global write "Verbal.vi" "P3右"(w493) -> ()
            n250 = global write "Verbal.vi" "pz0?"(TRUE ("pz0?")) -> ()
            n251 = call "go_one_step.vi"("执行完毕"=w497, "error in"=w496, "Step"=w494, "Motor"=3, "CmdLib In"=w495) -> ()  [unwired: 1 in, 3 out]
          }
        }
      }
      event "坐标移动": Value Change {
        # "位置坐标是mm/um\n需要转换成步数"
        n252 = event-data() -> ("CtlRef"=w519:refnum<vi>, "OldVal"=w518:bool)  [unwired: 1 in, 4 out]
        n253 = global read "Verbal.vi" "位置"() -> (w517:dbl[][])
        n254 = call "KeyGray_normalbool.vi"("OldVal"=w518, "引用"=w519) -> ()  [unwired: 2 in]
        n255 = To Long Integer(number=w517) -> (32bit integer=w515:i32[][])
        n256 = local read "当前位置"() -> (w505:i32[])
        n257 = local read "坐标"() -> (w516:enum16{"位置0", "位置1", "位置2", "位置3"})
        n258 = local read "电机"() -> (w504:T1)
        n259 = Index Array(array=w515, index (row)=w504, index (col)=w516) -> (element=w508:i32)
        n260 = Index Array(array=w509, index=w504) -> (element=w507:dbl)
        n261 = Index Array(array=w505, index=w504) -> (element=w502:i32)
        n262 = Divide(x=w508, y=w507) -> (x/y=w506:dbl)
        n263 = To Long Integer(number=w506) -> (32bit integer=w503:i32)
        n264 = Greater Or Equal?(x=w503, y=w502) -> (x >= y?=w501:bool)
        n265 = case shown="\"大平台Z\"" w504 {
          tunnel: w503 -> [w521 w528 w532 w538 w546 w555]
          tunnel: w514 -> [w520 w527 w533 _ _ _]
          tunnel: w513 -> [w523 w526 w534 _ _ _]
          tunnel: w512 -> [w522 w525 w535 w541 w549 w557]
          tunnel: w511 -> [_ _ _ w540 w548 w556]
          tunnel: w510 -> [_ _ _ w539 w547 w554]
          tunnel: w501 -> [_ _ _ w537 w545 w553]
          frame "大平台X", Default {
            w524 = u8 0 items=["x", "y", "z"] ("motor")
            n266 = call "TMCM351-goJog.vi"("执行？"=w522, "错误输入"=w520, "step in"=w521, "motor"=w524, "com in"=w523) -> ()  [unwired: 2 in, 2 out]
          }
          frame "大平台Y" {
            w529 = u8 1 items=["x", "y", "z"] ("motor")
            n267 = call "TMCM351-goJog.vi"("执行？"=w525, "错误输入"=w527, "step in"=w528, "motor"=w529, "com in"=w526) -> ()  [unwired: 2 in, 2 out]
          }
          frame "大平台Z" {
            w536 = u8 2 items=["x", "y", "z"] ("motor")
            n268 = Multiply(x=w532, y=-1) -> (x*y=w530:i32)
            n269 = call "TMCM351-goJog.vi"("执行？"=w535, "错误输入"=w533, "step in"=w530, "motor"=w536, "com in"=w534) -> ()  [unwired: 2 in, 2 out]
          }
          frame "小平台X" {
            n270 = global write "Verbal.vi" "P1右"(w537) -> ()
            n271 = global read "Verbal.vi" "Device Address"() -> (w543:i32)
            n272 = global read "Verbal.vi" "DeviceKey"() -> (w544:string)
            n273 = call "AbsoluteMove.vi"("CmdLib In"=w540, "DeviceKey In"=w544, "Device Address In"=w543, "Motor"=1, "Target Pos"=w538, "error in (no error)"=w539, "执行"=w541) -> ()  [unwired: 9 in, 4 out]
          }
          frame "小平台Y" {
            n274 = global write "Verbal.vi" "P2右"(w545) -> ()
            n275 = global read "Verbal.vi" "Device Address"() -> (w551:i32)
            n276 = global read "Verbal.vi" "DeviceKey"() -> (w552:string)
            n277 = call "AbsoluteMove.vi"("CmdLib In"=w548, "DeviceKey In"=w552, "Device Address In"=w551, "Motor"=2, "Target Pos"=w546, "error in (no error)"=w547, "执行"=w549) -> ()  [unwired: 9 in, 4 out]
          }
          frame "小平台Z" {
            n278 = global write "Verbal.vi" "P3右"(w553) -> ()
            n279 = global read "Verbal.vi" "Device Address"() -> (w559:i32)
            n280 = global read "Verbal.vi" "DeviceKey"() -> (w560:string)
            n281 = call "AbsoluteMove.vi"("CmdLib In"=w556, "DeviceKey In"=w560, "Device Address In"=w559, "Motor"=3, "Target Pos"=w555, "error in (no error)"=w554, "执行"=w557) -> ()  [unwired: 9 in, 4 out]
          }
        }
      }
    }
    n282 = global read "Verbal.vi" "小平台X限位"() -> (w187:dbl)
    n283 = global read "Verbal.vi" "位置"() -> (w188:dbl[][])
    n284 = global read "Verbal.vi" "JogCSV路径"() -> (w186:path)
  }
  n285 = flat-sequence {
    tunnel: w15 -> [w571]
    tunnel: w14 -> [w570]
    tunnel: w13 -> [w569]
    tunnel: w12 -> [w568]
    tunnel: w11 -> [w567]
    tunnel: w10 -> [w565]
    tunnel: w9 -> [w564]
    tunnel: w5 -> [w562]
    tunnel: w1 -> [w561]
    frame #0 {
      n286 = call "StopAll.vi"("StepError"=w567, "PicError"=w569, "com in"=w568, "CmdLib In"=w570) -> ("错误输出"=w566:errorcluster)
      n287 = Release Queue(queue=w571, error in (no error)=w566) -> (error out=w563:errorcluster)  [unwired: 1 in, 2 out]
      n288 = call "Write_lastpoint.vi"("Jog.csv"=w561, "坐标位置"=w565, "本次位置数据"=w562, "小平台X轴正限位mm"=w564, "error in (no error)"=w563) -> ()  [unwired: 1 in, 1 out]
    }
    frame #1 {
      n289 = Quit LabVIEW(quit? (T)=TRUE ("退出？(T)")) -> ()
    }
  }
